vi "robot_control.vi"(0 "Digital in":refnum<vi>, 1 "circle_state":i8, 2 "reference 3":refnum<vi>, 3 "Robot_vel":dbl, 4 "reference 4":refnum<vi>, 5 "go home":bool, 6 "reference 5":refnum<vi>, 8 "reference in":refnum<vi>, 9 "reference 6":refnum<vi>, 10 "Next point in circle":bool, 11 "reference 7":refnum<vi>, 12 "circle number of points":i8, 13 "Robot_connection":refnum<k5>, 14 "circle_radius (mm)":dbl, 15 "previous":bool, 16 "Robot_acc":dbl) -> ()   [LabVIEW 2024]
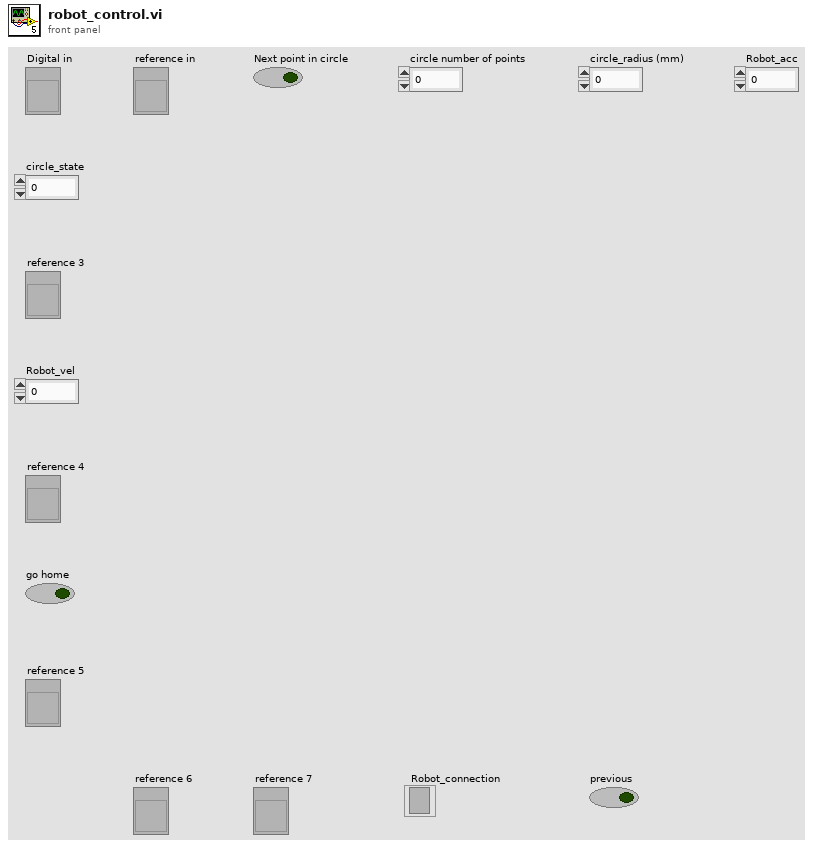
[diagram p1: front panel]
types:
  T1 = cluster{"Focus routine":bool, "Freedrive mode":bool, "Next point in circle":bool, "previous":bool, "go home":bool}
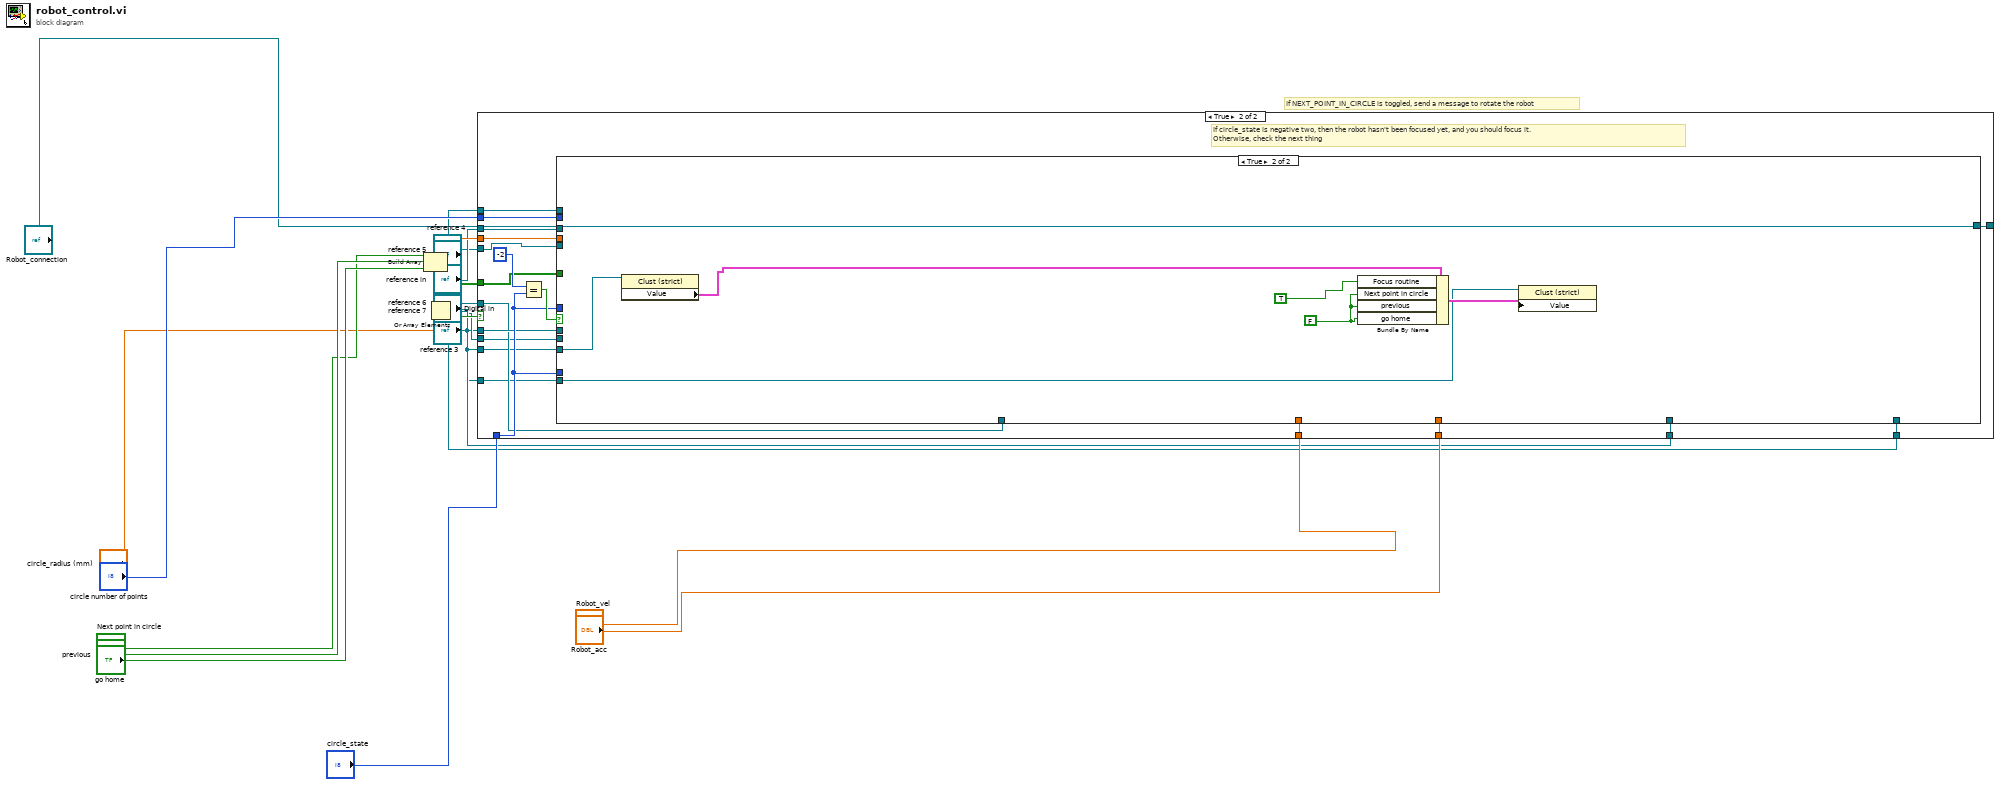
[diagram p0: block diagram]
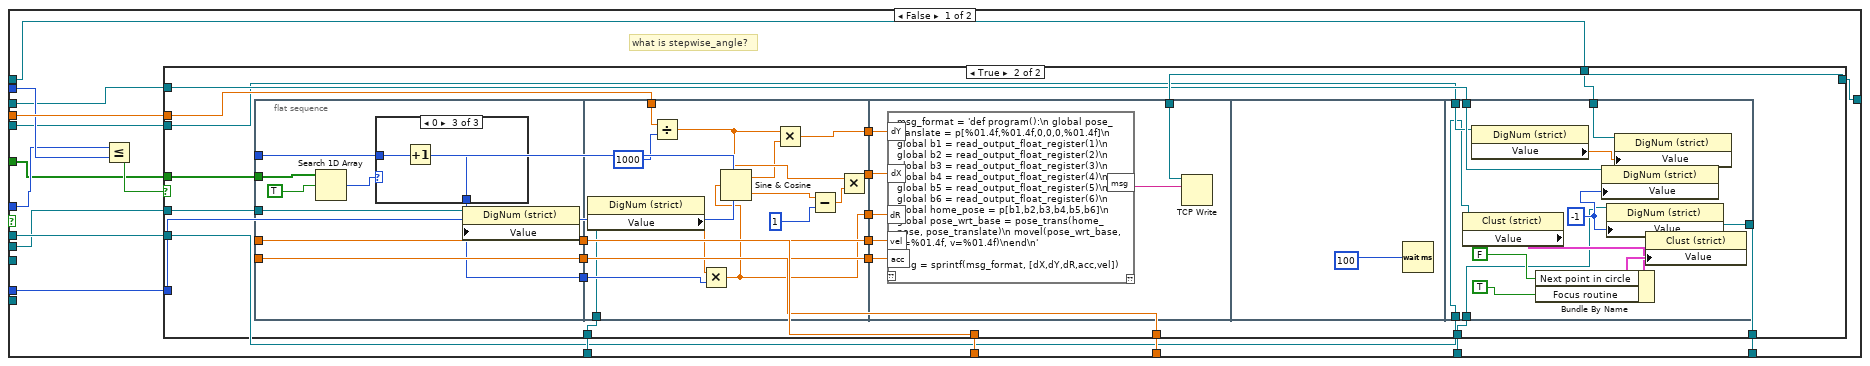
[diagram p3: hidden frame]
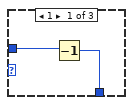
[diagram p5: hidden frame]
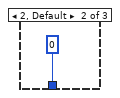
[diagram p6: hidden frame]
diagram:
  # "If NEXT_POINT_IN_CIRCLE is toggled, send a message to rotate the robot"
  n1 = Build Array("Next point in circle", "previous", "go home") -> (w18:bool[])
  n2 = Or Array Elements(Boolean array=w18) -> (logical OR=w17:bool)
  n3 = case shown="True" w17 {
    tunnel: "circle_state" -> [_ w32]
    tunnel: "circle number of points" -> [_ w35]
    tunnel: "Robot_vel" -> [_ w34]
    tunnel: "Robot_acc" -> [_ w33]
    tunnel: "circle_radius (mm)" -> [_ w31]
    tunnel: "Robot_connection" -> [_ w30]
    tunnel: w18 -> [_ w29]
    tunnel: "Digital in" -> [_ w28]
    tunnel: "reference in" -> [_ w27]
    tunnel: "reference 3" -> [_ w26]
    tunnel: "reference 4" -> [_ w25]
    tunnel: "reference 5" -> [_ w24]
    tunnel: "reference 3" -> [_ w23]
    tunnel: "reference 6" -> [_ w22]
    tunnel: "reference 7" -> [_ w21]
    tunnel: "reference 3" -> [_ w20]
    tunnel: "reference 3" -> [_ w19]
    frame False {
    }
    frame True {
      # "If circle_state is negative two, then the robot hasn't been focused yet, and you should focus it.\nOtherwise, check the next thing"
      n4 = Equal?(x=-2, y=w32) -> (x = y?=w36:bool)
      n5 = case shown="False" w36 {
        tunnel: w35 -> [w49 _]
        tunnel: w32 -> [w48 _]
        tunnel: w34 -> [w54 _]
        tunnel: w33 -> [w53 _]
        tunnel: w32 -> [w52 _]
        tunnel: w31 -> [w51 _]
        tunnel: w30 -> [w50 _]
        tunnel: w29 -> [w46 _]
        tunnel: w28 -> [w45 _]
        tunnel: w27 -> [w44 _]
        tunnel: w26 -> [w43 _]
        tunnel: w25 -> [w42 _]
        tunnel: w24 -> [w41 _]
        tunnel: w23 -> [w40 _]
        tunnel: w22 -> [w39 _]
        tunnel: w21 -> [w38 _]
        tunnel: w20 -> [_ w126]
        tunnel: w19 -> [_ w125]
        frame False {
          # "what is stepwise_angle?"
          n6 = Less Or Equal?(x=w48, y=w49) -> (x <= y?=w47:bool)
          n7 = case shown="True" w47 {
            tunnel: w54 -> [_ w76]
            tunnel: w53 -> [_ w75]
            tunnel: w52 -> [_ w65]
            tunnel: w51 -> [_ w66]
            tunnel: w50 -> [_ w74]
            tunnel: w46 -> [_ w63]
            tunnel: w45 -> [_ w62]
            tunnel: w44 -> [_ w61]
            tunnel: w43 -> [_ w60]
            tunnel: w42 -> [_ w59]
            tunnel: w41 -> [_ w58]
            tunnel: w40 -> [_ w57]
            tunnel: w39 -> [_ w56]
            tunnel: w38 -> [_ w55]
            frame False {
            }
            frame True {
              n8 = flat-sequence {
                tunnel: w65 -> [w82]
                tunnel: w75 -> [w83]
                tunnel: w76 -> [w84]
                tunnel: [w84] -> w68
                tunnel: [w83] -> w67
                tunnel: [w78] -> w64
                tunnel: w63 -> [w81]
                tunnel: w55 -> [w77]
                tunnel: [w104] -> w73
                tunnel: [w103] -> w72
                tunnel: [w92] -> w71
                tunnel: [w93] -> w70
                tunnel: [w94] -> w69
                tunnel: w68 -> [w104]
                tunnel: w67 -> [w103]
                tunnel: w66 -> [w96]
                tunnel: w64 -> [w91]
                tunnel: w56 -> [w90]
                tunnel: w74 -> [w105]
                tunnel: w73 -> [w111]
                tunnel: w72 -> [w110]
                tunnel: w71 -> [w109]
                tunnel: w70 -> [w108]
                tunnel: w69 -> [w107]
                tunnel: w62 -> [w118]
                tunnel: w61 -> [w117]
                tunnel: w60 -> [w116]
                tunnel: w59 -> [w115]
                tunnel: w58 -> [w114]
                tunnel: w57 -> [w113]
                frame #0 {
                  n9 = Search 1D Array(1D array=w81, element=TRUE) -> (index of element=w79:i32)  [unwired: 1 in]
                  n10 = case shown="0" w79 {
                    tunnel: w82 -> [w86 _ w89]
                    tunnel: [w85 0 w88] -> w78
                    frame 1 {
                      n11 = Decrement(x=w86) -> (x-1=w85:i8)
                    }
                    frame 2, Default {
                    }
                    frame 0 {
                      n12 = Increment(x=w89) -> (x+1=w88:i8)
                    }
                  }
                  n13 = property class="DigNum (strict)"(reference=w77, "Value"=w78) -> ()  [unwired: 1 in, 2 out]
                }
                frame #1 {
                  n14 = property class="DigNum (strict)"(reference=w90) -> ("Value"=w98:dbl)  [unwired: 1 in, 2 out]
                  n15 = Divide(x=w96, y=1000) -> (x/y=w101:dbl)
                  n16 = Multiply(x=w98, y=w91) -> (x*y=w92:dbl)
                  n17 = Sine & Cosine(0:w92) -> (1:w99:dbl, 2:w102:dbl)
                  n18 = Multiply(x=w101, y=w99) -> (x*y=w93:dbl)
                  n19 = Subtract(x=w102, y=1) -> (x-y=w100:dbl)
                  n20 = Multiply(x=w101, y=w100) -> (x*y=w94:dbl)
                }
                frame #2 {
                  n21 = script code="msg_format = 'def program():\\n global pose_translate = p[%01.4f,%01.4f,0,0,0,%01.4f]\\n global b1 = read_output_float_register(1)\\n global b2 = read_output_float_register(2)\\n global b3 = read_output_float_register(3)\\n global b4 = read_output_float_register(4)\\n global b5 = read_output_float_register(5)\\n global b6 = read_output_float_register(6)\\n global home_pose = p[b1,b2,b3,b4,b5,b6]\\n global pose_wrt_base = pose_trans(home_pose, pose_translate)\\n movel(pose_wrt_base, a=%01.4f, v=%01.4f)\\nend\\n'\n\nmsg = sprintf(msg_format, [dX,dY,dR,acc,vel])"("dX"=w107, "dY"=w108, "dR"=w109, "vel"=w111, "acc"=w110) -> ("msg"=w106:string)  [unwired: 1 in, 1 out]
                  n22 = TCP Write(connection ID=w105, data in=w106) -> ()  [unwired: 2 in, 3 out]
                }
                frame #3 {
                  n23 = Wait (ms)(milliseconds to wait=100) -> ()  [unwired: 1 out]
                }
                frame #4 {
                  w124 = -1
                  n24 = property class="Clust (strict)"(reference=w113) -> ("Value"=w121:T1)  [unwired: 1 in, 2 out]
                  n25 = property class="DigNum (strict)"(reference=w114) -> ("Value"=w123:dbl)  [unwired: 1 in, 2 out]
                  n26 = Bundle By Name(cluster=w121, "Next point in circle"=FALSE, "Focus routine"=TRUE) -> (w122:T1)
                  n27 = property class="DigNum (strict)"(reference=w117, "Value"=w124) -> ()  [unwired: 1 in, 2 out]
                  n28 = property class="DigNum (strict)"(reference=w118, "Value"=w124) -> ()  [unwired: 1 in, 2 out]
                  n29 = property class="DigNum (strict)"(reference=w115, "Value"=w123) -> ()  [unwired: 1 in, 2 out]
                  n30 = property class="Clust (strict)"(reference=w116, "Value"=w122) -> ()  [unwired: 1 in, 2 out]
                }
              }
            }
          }
        }
        frame True {
          w127 = FALSE
          n31 = property class="Clust (strict)"(reference=w125) -> ("Value"=w128:T1)  [unwired: 1 in, 2 out]
          n32 = Bundle By Name(cluster=w128, "Focus routine"=TRUE, "Next point in circle"=w127, "previous"=w127, "go home"=w127) -> (w129:T1)
          n33 = property class="Clust (strict)"(reference=w126, "Value"=w129) -> ()  [unwired: 1 in, 2 out]
        }
      }
    }
  }
